vi "updateStatesQueue.vi"(4 "States Updates":T1[](array[typedef]), 6 "State Queue Options":enum16{"Replace", "Append", "Prepend"}(ring)=enum."Append", 8 "error in (no error)":errorcluster, 11 "guiTemplates in":refnum<class "stillnessHelper.lvclass">) -> (0 "error out":errorcluster, 3 "guiTemplates out":refnum<class "stillnessHelper.lvclass">)   [LabVIEW 2022 SP3, in "stillnessHelper.lvclass"]
uses:
  stillnessHelper.lvclass
  stillnessHelper.lvclass/stillnessHelper.ctl
  statesWithOptions.ctl
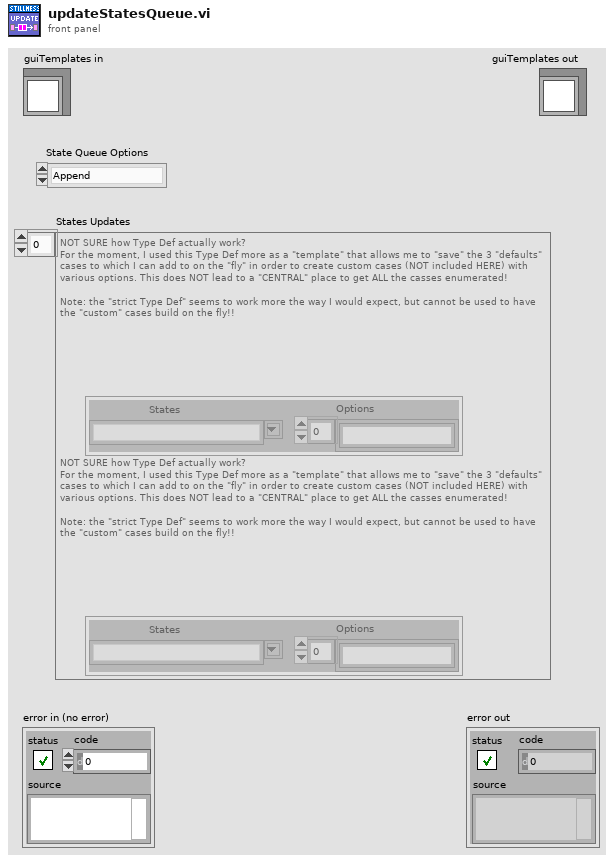
[diagram p1: front panel]
types:
  T1 = typedef "stillnessHelper.lvclass/statesWithOptions.ctl" = cluster{"States":string, "Options":string[]}
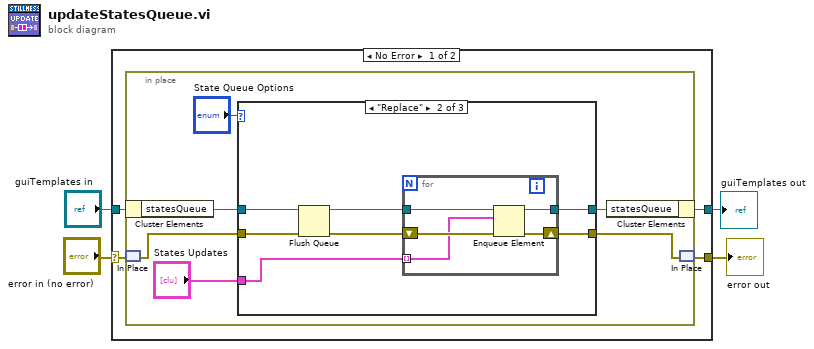
[diagram p0: block diagram]
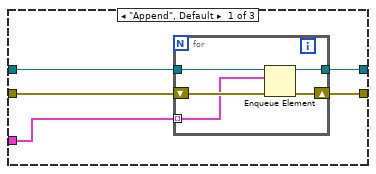
[diagram p2: hidden frame]
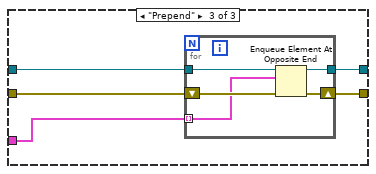
[diagram p3: hidden frame]
diagram:
  n1 = case shown="No Error" "error in (no error)" {
    selector: "error in (no error)" -> [w6 w48]
    tunnel: [w5 w48] -> w3
    tunnel: [w7 w47] -> w1
    tunnel: "guiTemplates in" -> [w8 w47]
    frame No Error {
      n2 = in-place {
        n3 = in-place-cluster #1(w8) -> ("statesQueue"=w13:refnum<queue>)
        n4 = in-place-match #2(w6) -> (w11:errorcluster)
        n5 = case shown="\"Replace\"" "State Queue Options" {
          tunnel: [w18 w31 w40] -> w12
          tunnel: "States Updates" -> [w16 w30 w38]
          tunnel: w13 -> [w19 w28 w41]
          tunnel: w11 -> [w17 w27 w39]
          tunnel: [w15 w29 w37] -> w10
          frame "Append", Default {
            n6 = for {
              shift-right: [w21] -> w15
              shift-left: w17 -> [w22]
              tunnel: w19 -> [w24]
              tunnel: [w23] -> w18
              tunnel: w16 -> [w20] mode=indexing
              n7 = Enqueue Element(queue=w24, element=w20, error in (no error)=w22) -> (queue out=w23:refnum<queue>, error out=w21:errorcluster)  [unwired: 1 in, 1 out]
            }
          }
          frame "Replace" {
            n8 = Flush Queue(queue=w28, error in (no error)=w27) -> (queue out=w25:refnum<queue>, error out=w26:errorcluster)  [unwired: 1 out]
            n9 = for {
              shift-right: [w33] -> w29
              shift-left: w26 -> [w34]
              tunnel: w25 -> [w36]
              tunnel: [w35] -> w31
              tunnel: w30 -> [w32] mode=indexing
              n10 = Enqueue Element(queue=w36, element=w32, error in (no error)=w34) -> (queue out=w35:refnum<queue>, error out=w33:errorcluster)  [unwired: 1 in, 1 out]
            }
          }
          frame "Prepend" {
            n11 = for {
              shift-right: [w43] -> w37
              shift-left: w39 -> [w44]
              tunnel: w41 -> [w46]
              tunnel: [w45] -> w40
              tunnel: w38 -> [w42] mode=indexing
              n12 = Enqueue Element At Opposite End(queue=w46, element=w42, error in (no error)=w44) -> (queue out=w45:refnum<queue>, error out=w43:errorcluster)  [unwired: 1 in, 1 out]
            }
          }
        }
        n13 = in-place-cluster #1("statesQueue"=w12) -> (w7:refnum<class "stillnessHelper.lvclass">)
        n14 = in-place-match #2(w10) -> (w5:errorcluster)
      }
    }
    frame Error {
    }
  }
  "error out" <- w3
  "guiTemplates out" <- w1
